vi "uActor_PreInit.vi"(8 "error in (no error)":errorcluster, 11 "uActor in":refnum<class "uActor.lvclass">) -> (0 "error out":errorcluster, 3 "uActor out":refnum<class "uActor.lvclass">)   [LabVIEW 2023, in "uFramework.lvlib" / "uActor.lvclass"]
doc: "Dynamic dispatch method that is called upstream the actor core method. This allows children to override the pre-initialization behavior. It is used when the helper loops in the actor core method requires preinitialization prior to calling the actor core."
uses:
  uActor.lvclass
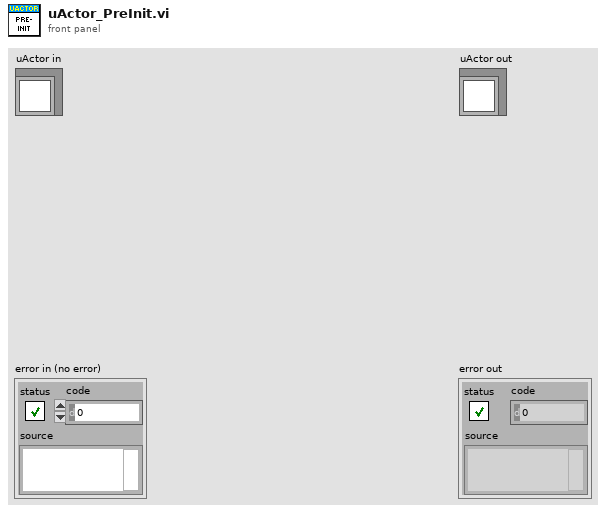
[diagram p1: front panel]
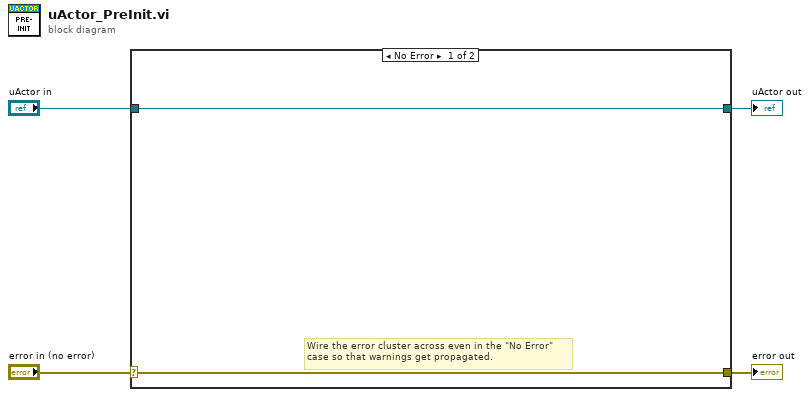
[diagram p0: block diagram]
diagram:
  n1 = case shown="No Error" "error in (no error)" {
    selector: "error in (no error)" -> [w5 w8]
    tunnel: [w5 w8] -> w3
    tunnel: [w6 w7] -> w1
    tunnel: "uActor in" -> [w6 w7]
    frame No Error {
      # "Wire the error cluster across even in the \"No Error\"\ncase so that warnings get propagated."
    }
    frame Error {
    }
  }
  "error out" <- w3
  "uActor out" <- w1
